vi "Hardware Device Get Info.vi"(8 "error in":errorcluster, 11 "NI Analog Output in":refnum<class "NI Analog Output.lvclass">) -> (0 "error out":errorcluster, 3 "NI Analog Output out":refnum<class "NI Analog Output.lvclass">)   [LabVIEW 2023, in "HardwareAbstractionLayer_LVOOP.lvlib" / "NI Analog Output.lvclass"]
doc: "This VI Device Physical Channel Read"
uses:
  NI Analog Output.lvclass
  NI Analog Output.lvclass/NI Analog Output.ctl
  <resource>/objmgr/daqmx.rc
  Teststand/Teststand.lvclass
panel:
  out "AO.PhysicalChans":tag[](array[tag])
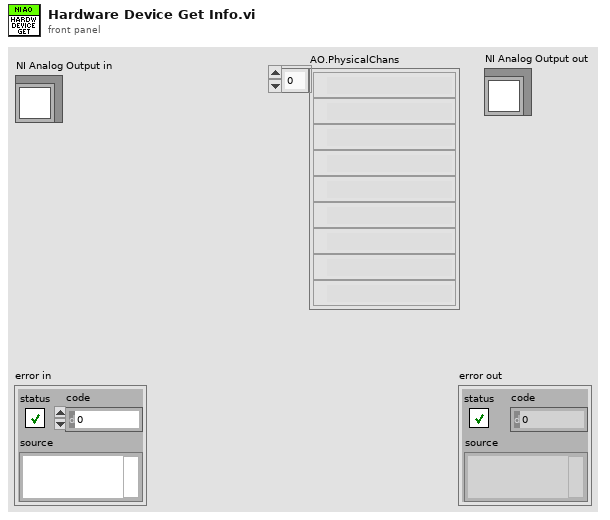
[diagram p1: front panel]
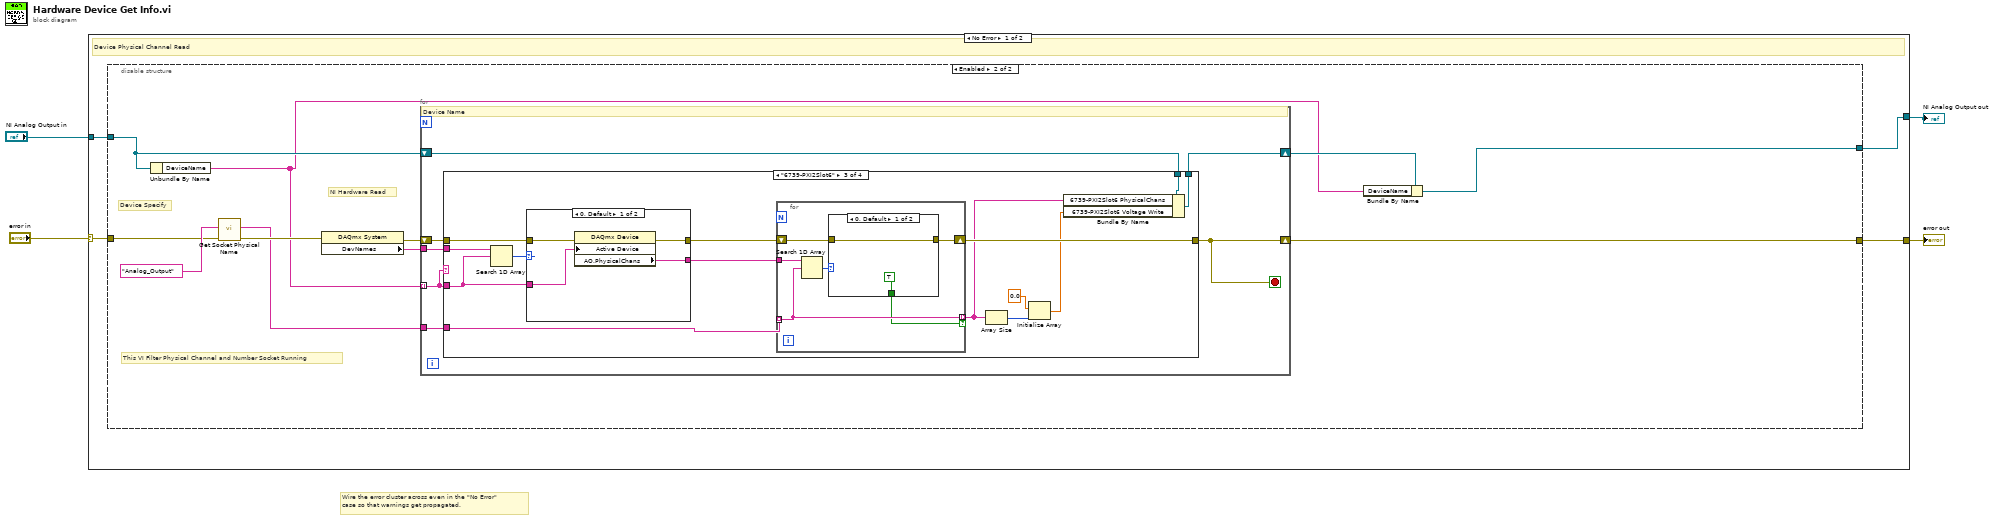
[diagram p0: block diagram]
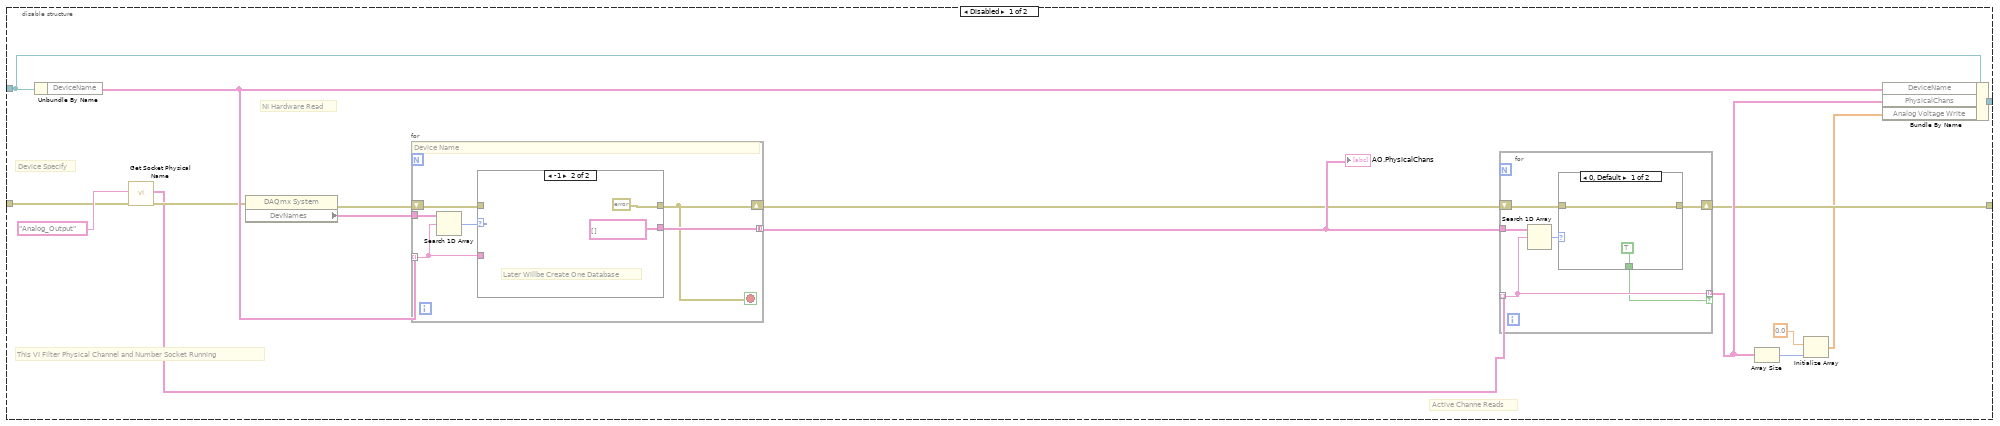
[diagram p2: hidden frame]
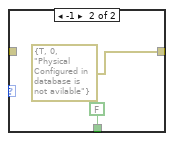
[diagram p3: hidden frame]
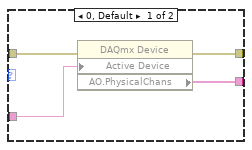
[diagram p4: hidden frame]
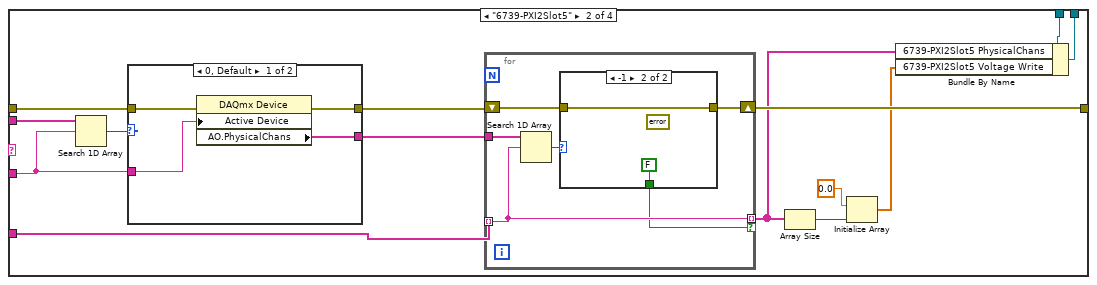
[diagram p6: hidden frame]
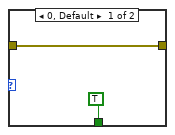
[diagram p7: hidden frame]
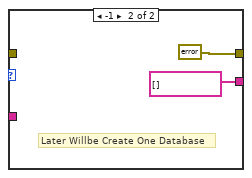
[diagram p8: hidden frame]
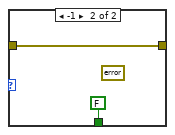
[diagram p9: hidden frame]
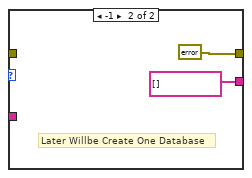
[diagram p10: hidden frame]
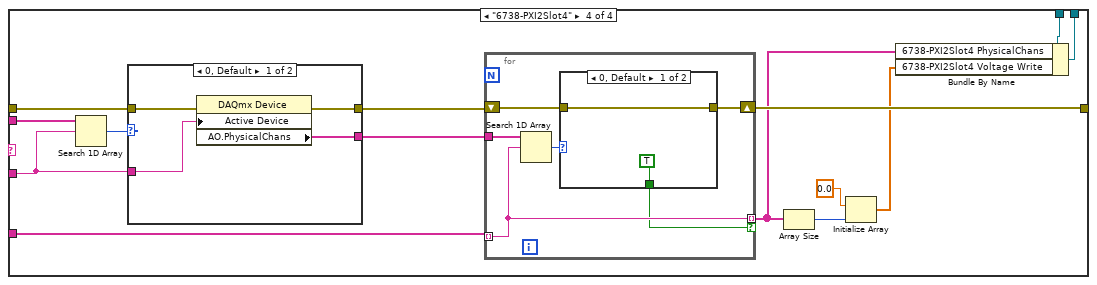
[diagram p11: hidden frame]
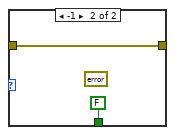
[diagram p12: hidden frame]
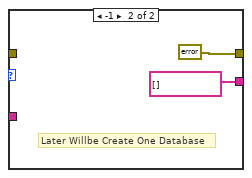
[diagram p13: hidden frame]
diagram:
  # "Wire the error cluster across even in the \"No Error\"\ncase so that warnings get propagated."
  n1 = case shown="No Error" "error in" {
    selector: "error in" -> [w6 w158]
    tunnel: [w5 w158] -> w3
    tunnel: [w8 w157] -> w1
    tunnel: "NI Analog Output in" -> [w7 w157]
    frame No Error {
      # "Device Physical Channel Read"
      n2 = disable-structure shown="Enabled" {
        disable-tunnel: [w19 w48] -> w8
        disable-tunnel: w7 -> [w18 w51]
        disable-tunnel: w6 -> [w13 w53]
        disable-tunnel: [w10 w50] -> w5
        frame Disabled {
          # "This VI Filter Physical Channel and Number Socket Running"
          # "Active Channe Reads"
          # "Device Specify"
          # "NI Hardware Read"
          n3 = Unbundle By Name(w18) -> ("DeviceName"=w24:tag[])
          n4 = call "Get Socket Physical Name.vi"("error In"=w13, "ChannelType"="Analog_Output") -> ("error out"=w12:errorcluster, "Physical Channel"=w11:tag[])  [unwired: 7 in, 1 out]
          n5 = property class="DAQmx System"(error in=w12) -> (error out=w22:errorcluster, "DevNames"=w23:tag[])  [unwired: 1 in, 1 out]
          n6 = for {
            tunnel: w24 -> [w37] mode=indexing
            tunnel: w23 -> [w38]
            tunnel: [w36] -> w21 mode=concatenating
            shift-right: [w35] -> w20
            shift-left: w22 -> [w39]
            stop <- w35 stop-if-true
            # "Device Name"
            n7 = Search 1D Array(1D array=w38, element=w37) -> (index of element=w40:i32)  [unwired: 1 in]
            n8 = case shown="-1" w40 {
              tunnel: w39 -> [w42 _]
              tunnel: [w41 errorcluster {"status"=TRUE, "code"=0, "source"="Device  Configured in database is not avilable"} ("error out")] -> w35
              tunnel: w37 -> [w44 _]
              tunnel: [w43 tag[] [] ("AI.PhysicalChans")] -> w36
              frame 0, Default {
                n9 = property class="DAQmx Device"(error in=w42, "Active Device"=w44) -> (error out=w41:errorcluster, "AO.PhysicalChans"=w43:tag[])  [unwired: 1 in, 1 out]
              }
              frame -1 {
                # "Later Willbe Create One Database"
              }
            }
          }
          "AO.PhysicalChans" <- w21
          n10 = for {
            tunnel: w21 -> [w30]
            tunnel: w11 -> [w26] mode=indexing
            shift-right: [w27] -> w10
            shift-left: w20 -> [w28]
            tunnel: [w26] -> w17 mode=indexing if=w25
            n11 = Search 1D Array(1D array=w30, element=w26) -> (index of element=w29:i32)  [unwired: 1 in]
            n12 = case shown="0, Default" w29 {
              tunnel: w28 -> [w32 _]
              tunnel: [w32 errorcluster {"status"=TRUE, "code"=0, "source"="Physical Configured in database is not avilable"} ("error out")] -> w27
              tunnel: [TRUE FALSE] -> w25
              frame 0, Default {
              }
              frame -1 {
              }
            }
          }
          n13 = Array Size(array=w17) -> (size(s)=w16:i32)
          n14 = Initialize Array(0.0, w16) -> (w9:dbl[])
          n15 = Bundle By Name(cluster=w18, "DeviceName"=w24, "PhysicalChans"=w17, "Analog Voltage Write"=w9) -> (w19:refnum<class "NI Analog Output.lvclass">)
        }
        frame Enabled {
          # "This VI Filter Physical Channel and Number Socket Running"
          # "Device Specify"
          # "NI Hardware Read"
          n16 = Unbundle By Name(w51) -> ("DeviceName"=w47:tag[])
          n17 = call "Get Socket Physical Name.vi"("error In"=w53, "ChannelType"="Analog_Output") -> ("error out"=w55:errorcluster, "Physical Channel"=w52:tag[])  [unwired: 7 in, 1 out]
          n18 = property class="DAQmx System"(error in=w55) -> (error out=w56:errorcluster, "DevNames"=w57:tag[])  [unwired: 1 in, 1 out]
          n19 = for {
            tunnel: w47 -> [w61] mode=indexing
            tunnel: w57 -> [w63]
            shift-right: [w62] -> w50
            shift-left: w56 -> [w64]
            tunnel: w52 -> [w60]
            shift-right: [w58] -> w49
            shift-left: w51 -> [w59]
            stop <- w62 stop-if-true
            # "Device Name"
            n20 = case shown="\"6739-PXI2Slot6\"" w61 {
              tunnel: w64 -> [w65 w79 w109 w139]
              tunnel: w63 -> [_ w67 w97 w127]
              tunnel: w61 -> [_ w78 w108 w138]
              tunnel: [w65 w76 w106 w136] -> w62
              tunnel: w60 -> [_ w74 w104 w134]
              tunnel: w59 -> [w66 w71 w101 w131]
              tunnel: [w66 w70 w100 w130] -> w58
              frame "", Default {
              }
              frame "6739-PXI2Slot5" {
                n21 = Search 1D Array(1D array=w67, element=w78) -> (index of element=w80:i32)  [unwired: 1 in]
                n22 = case shown="0, Default" w80 {
                  tunnel: w79 -> [w92 _]
                  tunnel: [w91 errorcluster {"status"=TRUE, "code"=0, "source"="Device  Configured in database is not avilable"} ("error out")] -> w77
                  tunnel: w78 -> [w94 _]
                  tunnel: [w93 tag[] [] ("AI.PhysicalChans")] -> w75
                  frame 0, Default {
                    n23 = property class="DAQmx Device"(error in=w92, "Active Device"=w94) -> (error out=w91:errorcluster, "AO.PhysicalChans"=w93:tag[])  [unwired: 1 in, 1 out]
                  }
                  frame -1 {
                    # "Later Willbe Create One Database"
                  }
                }
                n24 = for {
                  tunnel: w75 -> [w86]
                  tunnel: w74 -> [w82] mode=indexing
                  shift-right: [w83] -> w76
                  shift-left: w77 -> [w84]
                  tunnel: [w82] -> w68 mode=indexing if=w81
                  n25 = Search 1D Array(1D array=w86, element=w82) -> (index of element=w85:i32)  [unwired: 1 in]
                  n26 = case shown="-1" w85 {
                    tunnel: w84 -> [w88 w89]
                    tunnel: [w88 w89] -> w83
                    tunnel: [TRUE FALSE] -> w81
                    frame 0, Default {
                    }
                    frame -1 {
                      (unwired) errorcluster {"status"=TRUE, "code"=0, "source"="Physical Configured in database is not avilable"} ("error out")
                    }
                  }
                }
                n27 = Array Size(array=w68) -> (size(s)=w72:i32)
                n28 = Initialize Array(0.0, w72) -> (w69:dbl[])
                n29 = Bundle By Name(cluster=w71, "6739-PXI2Slot5 PhysicalChans"=w68, "6739-PXI2Slot5 Voltage Write"=w69) -> (w70:refnum<class "NI Analog Output.lvclass">)
              }
              frame "6739-PXI2Slot6" {
                n30 = Search 1D Array(1D array=w97, element=w108) -> (index of element=w110:i32)  [unwired: 1 in]
                n31 = case shown="0, Default" w110 {
                  tunnel: w109 -> [w122 _]
                  tunnel: [w121 errorcluster {"status"=TRUE, "code"=0, "source"="Device  Configured in database is not avilable"} ("error out")] -> w107
                  tunnel: w108 -> [w124 _]
                  tunnel: [w123 tag[] [] ("AI.PhysicalChans")] -> w105
                  frame 0, Default {
                    n32 = property class="DAQmx Device"(error in=w122, "Active Device"=w124) -> (error out=w121:errorcluster, "AO.PhysicalChans"=w123:tag[])  [unwired: 1 in, 1 out]
                  }
                  frame -1 {
                    # "Later Willbe Create One Database"
                  }
                }
                n33 = for {
                  tunnel: w105 -> [w116]
                  tunnel: w104 -> [w112] mode=indexing
                  shift-right: [w113] -> w106
                  shift-left: w107 -> [w114]
                  tunnel: [w112] -> w98 mode=indexing if=w111
                  n34 = Search 1D Array(1D array=w116, element=w112) -> (index of element=w115:i32)  [unwired: 1 in]
                  n35 = case shown="0, Default" w115 {
                    tunnel: w114 -> [w118 w119]
                    tunnel: [w118 w119] -> w113
                    tunnel: [TRUE FALSE] -> w111
                    frame 0, Default {
                    }
                    frame -1 {
                      (unwired) errorcluster {"status"=TRUE, "code"=0, "source"="Physical Configured in database is not avilable"} ("error out")
                    }
                  }
                }
                n36 = Array Size(array=w98) -> (size(s)=w102:i32)
                n37 = Initialize Array(0.0, w102) -> (w99:dbl[])
                n38 = Bundle By Name(cluster=w101, "6739-PXI2Slot6 PhysicalChans"=w98, "6739-PXI2Slot6 Voltage Write"=w99) -> (w100:refnum<class "NI Analog Output.lvclass">)
              }
              frame "6738-PXI2Slot4" {
                n39 = Search 1D Array(1D array=w127, element=w138) -> (index of element=w140:i32)  [unwired: 1 in]
                n40 = case shown="0, Default" w140 {
                  tunnel: w139 -> [w152 _]
                  tunnel: [w151 errorcluster {"status"=TRUE, "code"=0, "source"="Device  Configured in database is not avilable"} ("error out")] -> w137
                  tunnel: w138 -> [w154 _]
                  tunnel: [w153 tag[] [] ("AI.PhysicalChans")] -> w135
                  frame 0, Default {
                    n41 = property class="DAQmx Device"(error in=w152, "Active Device"=w154) -> (error out=w151:errorcluster, "AO.PhysicalChans"=w153:tag[])  [unwired: 1 in, 1 out]
                  }
                  frame -1 {
                    # "Later Willbe Create One Database"
                  }
                }
                n42 = for {
                  tunnel: w135 -> [w146]
                  tunnel: w134 -> [w142] mode=indexing
                  shift-right: [w143] -> w136
                  shift-left: w137 -> [w144]
                  tunnel: [w142] -> w128 mode=indexing if=w141
                  n43 = Search 1D Array(1D array=w146, element=w142) -> (index of element=w145:i32)  [unwired: 1 in]
                  n44 = case shown="0, Default" w145 {
                    tunnel: w144 -> [w148 w149]
                    tunnel: [w148 w149] -> w143
                    tunnel: [TRUE FALSE] -> w141
                    frame 0, Default {
                    }
                    frame -1 {
                      (unwired) errorcluster {"status"=TRUE, "code"=0, "source"="Physical Configured in database is not avilable"} ("error out")
                    }
                  }
                }
                n45 = Array Size(array=w128) -> (size(s)=w132:i32)
                n46 = Initialize Array(0.0, w132) -> (w129:dbl[])
                n47 = Bundle By Name(cluster=w131, "6738-PXI2Slot4 PhysicalChans"=w128, "6738-PXI2Slot4 Voltage Write"=w129) -> (w130:refnum<class "NI Analog Output.lvclass">)
              }
            }
          }
          n48 = Bundle By Name(cluster=w49, "DeviceName"=w47) -> (w48:refnum<class "NI Analog Output.lvclass">)
        }
      }
    }
    frame Error {
    }
  }
  "error out" <- w3
  "NI Analog Output out" <- w1
